vi "Drive Train.vi"   [LabVIEW 2018]
uses:
  <vilib>/Rock Robotics/SystemInterfaces/DIO/FPGA_DIOChannel.ctl
  <vilib>/Rock Robotics/SystemInterfaces/AI/FPGA_AIChannel.ctl
  <vilib>/Rock Robotics/WPI/ThirdParty/Sensors/navX/_TypeDefs/FRIC_navX_DeviceNumbersTypeDef.ctl
  <vilib>/Rock Robotics/WPI/ThirdParty/Phoenix-LabVIEW/Motor Controller/Controls/CTRE_Phoenix_MotorControl_NeutralMode.ctl
  <vilib>/Rock Robotics/WPI/Counter/WPI_CounterDigitalInputToDigitalSource.vi
  Times/Times Global.vi
  Drive Train Global.vi
types:
  T1 = typedef "FPGA_AIChannel.ctl" = enum8{"AI 0", "AI 1", "AI 2", "AI 3", "AI MXP 0", "AI MXP 1", "AI MXP 2", "AI MXP 3", "Invalid"}
  T2 = typedef "FPGA_DIOChannel.ctl" = enum8{"DIO 0", "DIO 1", "DIO 2", "DIO 3", "DIO 4", "DIO 5", "DIO 6", "DIO 7", "DIO 8", "DIO 9", "DIO MXP 0", "DIO MXP 1", "DIO MXP 2", "DIO MXP 3", "DIO MXP 4", "DIO MXP 5", "DIO MXP 6", "DIO MXP 7", "DIO MXP 8", "DIO MXP 9", "DIO MXP 10", "DIO MXP 11", "DIO MXP 12", "DIO MXP 13", "DIO MXP 14", "DIO MXP 15", "SPI Port CS1", "SPI Port CS2", "SPI Port CS3", "SPI Port MISO", "SPI Port MOSI", "Invalid"}
  T3 = typedef "CTRE_Phoenix_MotorControl_NeutralMode.ctl" = enum8{"EEPROMSetting", "Override to Coast", "Override to Brake"}
  T4 = typedef "WPI_MotorControlDeviceRef.ctl" = cluster{"DeviceStatus":errorcluster, "Type":T5, "PWM":cluster{"PWM Channel":T6, "DeadBand":T7}, "CAN":cluster{"Device Number":u8, "SetOutput VI Ref":variant, "GetOutput VI Ref":variant, "Enable VI Ref":variant, "Disable VI Ref":variant, "Data":variant}, "Invert":bool, "DIO PWM":cluster{"PWM \"Enable\" Channel":T6, "DIOChannel":T2, "PWM Rate":dbl}}
  T5 = typedef "WPI_MotorControlType.ctl" = enum16{"PWM", "CAN", "DIO PWM"}
  T6 = typedef "FPGA_DIOPWMChannel.ctl" = enum8{"PWM 0", "PWM 1", "PWM 2", "PWM 3", "PWM 4", "PWM 5", "PWM 6", "PWM 7", "PWM 8", "PWM 9", "PWM MXP 0", "PWM MXP 1", "PWM MXP 2", "PWM MXP 3", "PWM MXP 4", "PWM MXP 5", "PWM MXP 6", "PWM MXP 7", "PWM MXP 8", "PWM MXP 9", "Invalid"}
  T7 = typedef "WPI_PWMDeadband.ctl" = cluster{"Name":string, "maxPositivePwm":i32, "minPositivePwm":i32, "centerPwm":i32, "maxNegativePwm":i32, "minNegativePwm":i32, "angularRange":u16}
  T8 = typedef "WPI_DigitalInputDevRef.ctl" = cluster{"DevStatus":errorcluster, "DIO Channel":T2}
  T9 = typedef "WPI_PotentiometerDevRef.ctl" = cluster{"DevStatus":errorcluster, "Analog Channel":T1, "Invert Output":bool}
  T10 = typedef "FPGA_CounterEncoderSourceConvertionLVSourceType.ctl" = cluster{"DevStatus":errorcluster, "AnalogTriggerMode?":bool, "DigitalMode":cluster{"DIO Channel":T11}, "AnalogTriggerMode":cluster{"AnalogTriggerIndex":T12, "OutputType":T13}}
  T11 = typedef "FPGA_DIODigitalSourceChannel.ctl" = enum8{"DIO 0", "DIO 1", "DIO 2", "DIO 3", "DIO 4", "DIO 5", "DIO 6", "DIO 7", "DIO 8", "DIO 9", "DIO MXP 0", "DIO MXP 1", "DIO MXP 2", "DIO MXP 3", "DIO MXP 4", "DIO MXP 5", "DIO MXP 6", "DIO MXP 7", "DIO MXP 8", "DIO MXP 9", "DIO MXP 10", "DIO MXP 11", "DIO MXP 12", "DIO MXP 13", "DIO MXP 14", "DIO MXP 15", "SPI Port CS1", "SPI Port CS2", "SPI Port CS3", "SPI Port MISO", "SPI Port MOSI", "Disabled"}
  T12 = typedef "FPGA_AnalogTriggerIndex.ctl" = enum8{"Trig 0", "Trig 1", "Trig 2", "Trig 3", "Trig 4", "Trig 5", "Trig 6", "Trig 7", "Invalid"}
  T13 = typedef "FPGA_AnalogTriggerOutType.ctl" = enum16{"InWindow", "TriggerState", "Rising", "Falling"}
  T14 = typedef "WPI_EncoderDevRef.ctl" = cluster{"DevStatus":errorcluster, "EncoderIndex":T15, "CounterIndex":T16, "DistancePerCount":dbl, "Decoding Type":T17}
  T15 = typedef "FPGA_EncoderIdx.ctl" = enum8{"Enc 0", "Enc 1", "Enc 2", "Enc 3", "Enc 4", "Enc 5", "Enc 6", "Enc 7", "Invalid"}
  T16 = typedef "FPGA_CounterCtrSystemIndex.ctl" = enum8{"Ctr 0", "Ctr 1", "Ctr 2", "Ctr 3", "Ctr 4", "Ctr 5", "Ctr 6", "Ctr 7", "Invalid"}
  T17 = typedef "WPI_EncoderType.ctl" = enum16{"1x", "2x", "4x"}
  T18 = typedef "FRIC_navX_DeviceNumbersTypeDef.ctl" = enum16{"Dev0", "Dev1", "Dev2", "Dev3"}
  T19 = typedef "Control 2.ctl" = dbl
  T20 = cluster{"Rollover":dbl, "Yaw":dbl, "Cont Yaw":dbl}
  T21 = cluster{"FrontLeft":dbl, "FrontRight":dbl, "BackLeft":dbl, "BackRight":dbl}
  T22 = enum16{"Back Left", "Back Right", "Front Left", "Front Right"}
  T23 = enum16{"Autonomous Mode", "Field Oriented", "Robot Oriented", "Tank Mode"}
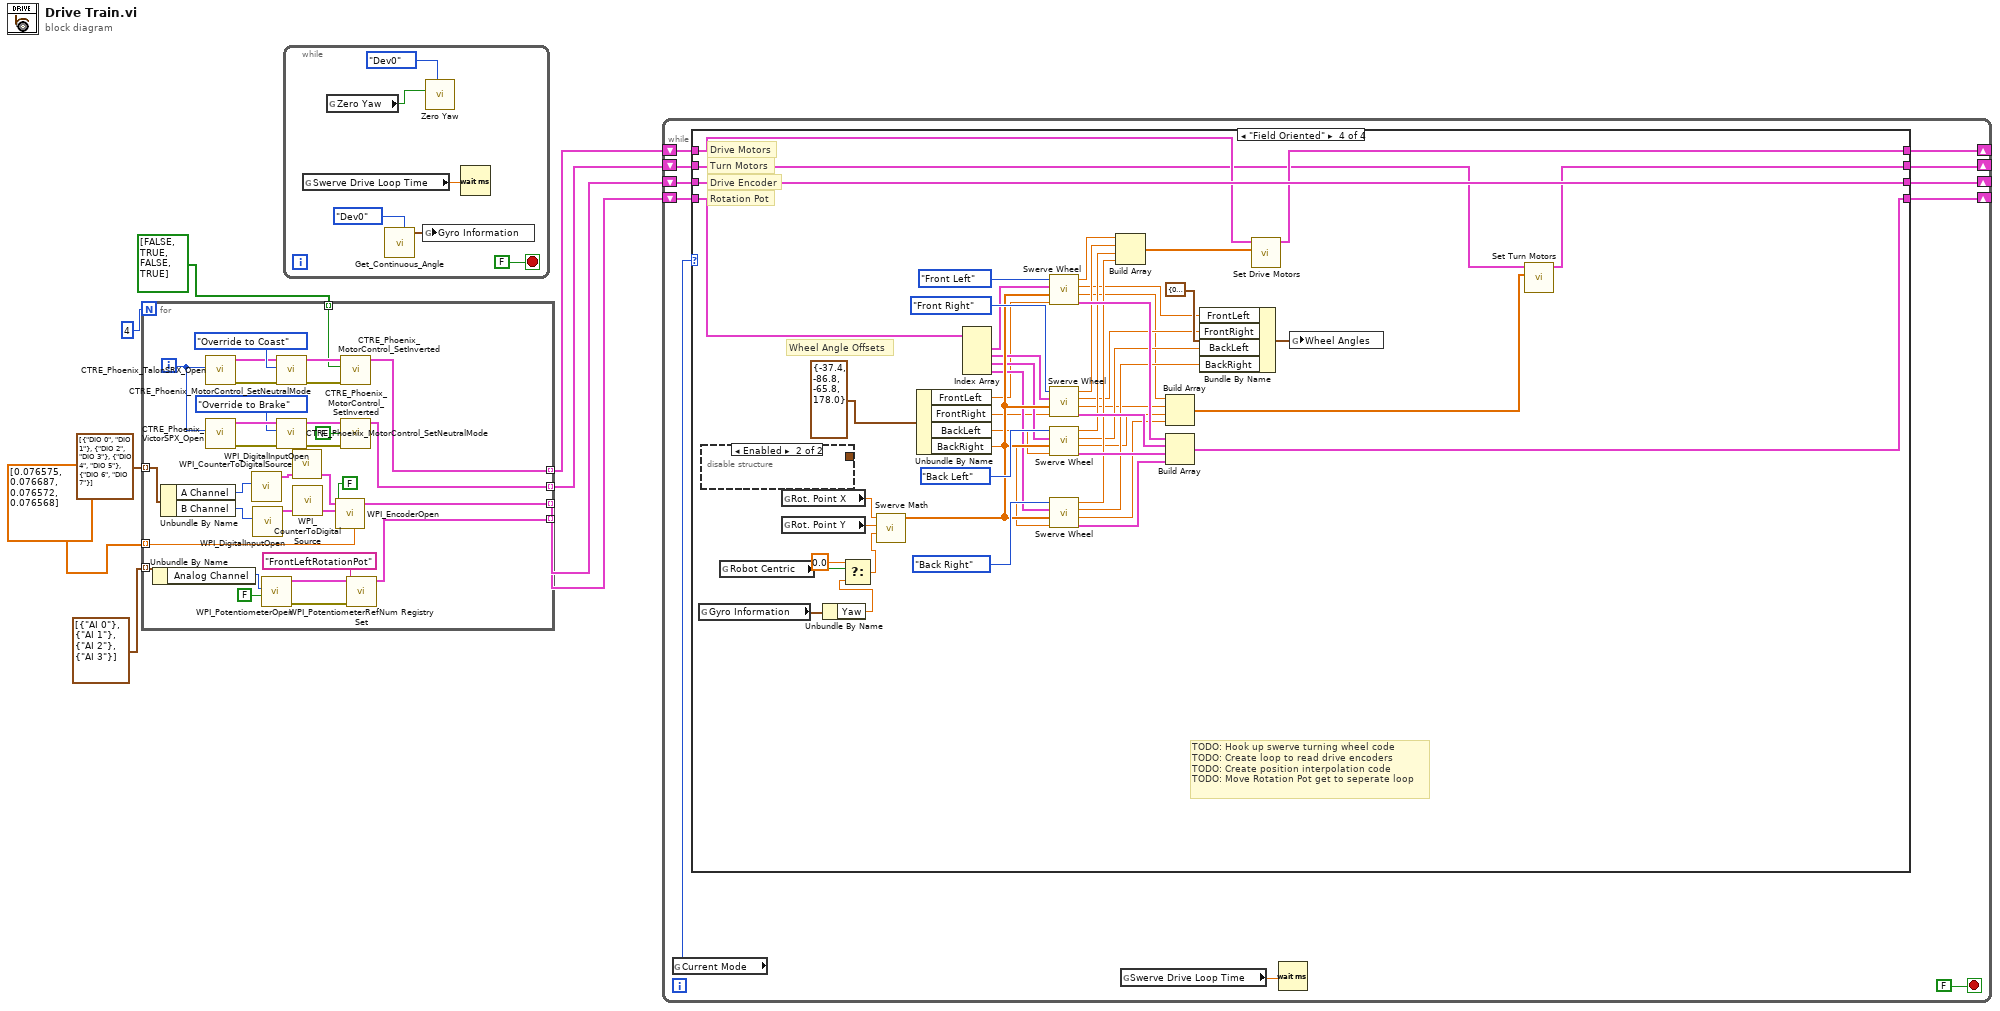
[diagram p0: block diagram]
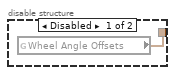
[diagram p5: hidden frame]
diagram:
  n1 = for {
    N: 4 -> [_]
    tunnel: cluster{"A Channel":T2, "B Channel":T2}[] [{"A Channel"=enum."DIO 0", "B Channel"=enum."DIO 1"}, {"A Channel"=enum."DIO 2", "B Channel"=enum."DIO 3"}, {"A Channel"=enum."DIO 4", "B Channel"=enum."DIO 5"}, {"A Channel"=enum."DIO 6", "B Channel"=enum."DIO 7"}] -> [w20] mode=indexing
    tunnel: cluster{"Analog Channel":T1}[] [{"Analog Channel"=enum."AI 0"}, {"Analog Channel"=enum."AI 1"}, {"Analog Channel"=enum."AI 2"}, {"Analog Channel"=enum."AI 3"}] -> [w17] mode=indexing
    tunnel: dbl[] [0.076575, 0.076687, 0.076572, 0.076568] -> [w15] mode=indexing
    tunnel: [w14] -> w5 mode=indexing
    tunnel: [w13] -> w4 mode=indexing
    tunnel: [w12] -> w3 mode=indexing
    tunnel: [w11] -> w2 mode=indexing
    tunnel: bool[] [FALSE, TRUE, FALSE, TRUE] -> [w10] mode=indexing
    i -> [w21]
    n2 = Unbundle By Name(w17) -> ("Analog Channel"=w16:T1)
    n3 = Unbundle By Name(w20) -> ("A Channel"=w19:T2, "B Channel"=w18:T2)
    n4 = call <vilib>:"CTRE_Phoenix_TalonSRX_Open.vi"("Device Number"=w21) -> ("error out"=w22:errorcluster, "CAN Talon SRX Ref"=w23:T4)  [unwired: 9 in]
    n5 = call <vilib>:"CTRE_Phoenix_VictorSPX_Open.vi"("Device Number"=w21) -> ("error out"=w32:errorcluster, "CAN Talon SRX Ref"=w31:T4)  [unwired: 9 in]
    n6 = call <vilib>:"WPI_DigitalInputOpen.vi"("DIO Channel"=w19) -> ("DigitalInputDevRef"=w39:T8)  [unwired: 1 in, 9 out]
    n7 = call <vilib>:"WPI_DigitalInputOpen.vi"("DIO Channel"=w18) -> ("DigitalInputDevRef"=w38:T8)  [unwired: 1 in, 9 out]
    n8 = call <vilib>:"WPI_PotentiometerOpen.vi"("Invert Output"=FALSE, "Analog Channel"=w16) -> ("error out"=w34:errorcluster, "PotDevRef"=w35:T9)  [unwired: 8 in]
    n9 = call <vilib>:"CTRE_Phoenix_MotorControl_SetNeutralMode.vi"("error in (no error)"=w22, "Motor Control Neutral Mode"=CTRE_Phoenix_MotorControl_NeutralMode."Override to Coast", "PhoenixMotorControlDevRef"=w23) -> ("error out"=w25:errorcluster, "PhoenixMotorControlDevRef"=w26:T4)  [unwired: 7 in]
    n10 = call <vilib>:"CTRE_Phoenix_MotorControl_SetNeutralMode.vi"("error in (no error)"=w32, "Motor Control Neutral Mode"=CTRE_Phoenix_MotorControl_NeutralMode."Override to Brake", "PhoenixMotorControlDevRef"=w31) -> ("error out"=w29:errorcluster, "PhoenixMotorControlDevRef"=w28:T4)  [unwired: 7 in]
    n11 = call-poly <vilib>:"WPI_CounterToDigitalSource.vi"("DigitalInputDevRef"=w39) -> ("Digital Source"=w40:T10)  [unwired: 6 out]
    n12 = call-poly <vilib>:"WPI_CounterToDigitalSource.vi"("DigitalInputDevRef"=w38) -> ("Digital Source"=w37:T10)  [unwired: 6 out]
    n13 = call <vilib>:"WPI_EncoderOpen.vi"("DistancePerCount"=w15, "Invert Direction (False)"=FALSE, "BSource"=w37, "ASource"=w40) -> ("EncoderDevRef"=w12:T14)  [unwired: 4 in, 3 out]
    n14 = call <vilib>:"CTRE_Phoenix_MotorControl_SetInverted.vi"("error in (no error)"=w25, "Invert?"=w10, "PhoenixMotorControlDevRef"=w26) -> ("PhoenixMotorControlDevRef"=w14:T4)  [unwired: 7 in, 1 out]
    n15 = call <vilib>:"CTRE_Phoenix_MotorControl_SetInverted.vi"("error in (no error)"=w29, "Invert?"=FALSE, "PhoenixMotorControlDevRef"=w28) -> ("PhoenixMotorControlDevRef"=w13:T4)  [unwired: 7 in, 1 out]
    n16 = call <vilib>:"WPI_PotentiometerRefNum Registry Set.vi"("error in (no error)"=w34, "refnum name"="FrontLeftRotationPot", "PotDevRef"=w35) -> ("PotDevRef"=w11:T9)  [unwired: 7 in, 1 out]
  }
  n17 = while {
    stop <- FALSE stop-if-true
    n18 = global read "Times Global.vi" "Swerve Drive Loop Time"() -> (w44:T19)
    n19 = global read "Drive Train Global.vi" "Zero Yaw"() -> (w43:bool)
    n20 = call <vilib>:"Get_Continuous_Angle.vi"("Device Number"=FRIC_navX_DeviceNumbersTypeDef."Dev0") -> ("Continuous Angle"=w45:T20)  [unwired: 10 in]
    n21 = global write "Drive Train Global.vi" "Gyro Information"(w45) -> ()
    n22 = call <vilib>:"Zero Yaw.vi"("Device Number"=FRIC_navX_DeviceNumbersTypeDef."Dev0", "Zero"=w43) -> ()  [unwired: 10 in]
    n23 = Wait (ms)(milliseconds to wait=w44) -> ()  [unwired: 1 out]
  }
  n24 = while {
    shift-right: [w51] -> _
    shift-left: w5 -> [w55]
    shift-right: [w50] -> _
    shift-left: w4 -> [w54]
    shift-right: [w49] -> _
    shift-left: w3 -> [w53]
    shift-right: [w48] -> _
    shift-left: w2 -> [w52]
    stop <- FALSE stop-if-true
    n25 = global read "Drive Train Global.vi" "Current Mode"() -> (w56:T23)
    n26 = case shown="\"Field Oriented\"" w56 {
      tunnel: w55 -> [w62 w66 w70 w94]
      tunnel: w54 -> [w61 w65 w69 w82]
      tunnel: w53 -> [w60 w64 w68 w114]
      tunnel: w52 -> [w59 w63 w67 w105]
      tunnel: [w62 w66 w70 w93] -> w51
      tunnel: [w61 w65 w69 w81] -> w50
      tunnel: [w60 w64 w68 w114] -> w49
      tunnel: [w59 w63 w67 w104] -> w48
      frame "Autonomous Mode", Default {
        # "Rotation Pot"
        # "Drive Encoder"
        # "Turn Motors"
        # "Drive Motors"
      }
      frame "Robot Oriented" {
        # "Rotation Pot"
        # "Drive Encoder"
        # "Turn Motors"
        # "Drive Motors"
      }
      frame "Tank Mode" {
        # "Rotation Pot"
        # "Drive Encoder"
        # "Turn Motors"
        # "Drive Motors"
      }
      frame "Field Oriented" {
        # "Wheel Angle Offsets"
        # "TODO: Hook up swerve turning wheel code\nTODO: Create loop to read drive encoders\nTODO: Create position interpolation code\nTODO: Move Rotation Pot get to seperate loop"
        # "Rotation Pot"
        # "Drive Encoder"
        # "Turn Motors"
        # "Drive Motors"
        n27 = global read "Drive Train Global.vi" "Gyro Information"() -> (w112:T20)
        n28 = disable-structure shown="Enabled" {
          disable-tunnel: [w119 _] -> _
          frame Disabled {
            n29 = global read "Drive Train Global.vi" "Wheel Angle Offsets"() -> (w119:T21)
          }
          frame Enabled {
          }
        }
        n30 = global read "Drive Train Global.vi" "Robot Centric"() -> (w74:bool)
        n31 = global read "Drive Train Global.vi" "Rot. Point X"() -> (w111:dbl)
        n32 = global read "Drive Train Global.vi" "Rot. Point Y"() -> (w110:dbl)
        n33 = Unbundle By Name(w112) -> ("Yaw"=w72:dbl)
        n34 = Select(t=0.0, s=w74, f=w72) -> (s? t:f=w75:dbl)
        n35 = call "Swerve Math.vi"("Yaw"=w75, "Rot. Point Y"=w110, "Rot. Point X"=w111) -> ("Swerve Math Ouput"=w113:dbl[])  [unwired: 8 in]
        n36 = Unbundle By Name(T21 {"FrontLeft"=-37.4, "FrontRight"=-86.8, "BackLeft"=-65.8, "BackRight"=178.0} ("Wheel Angle Offsets")) -> ("FrontLeft"=w79:dbl, "FrontRight"=w78:dbl, "BackLeft"=w77:dbl, "BackRight"=w76:dbl)
        n37 = Index Array(array=w105) -> (element #1=w109:T9, element #2=w108:T9, element #3=w107:T9, element #4=w106:T9)  [unwired: 4 in]
        n38 = call "Swerve Wheel.vi"("Wheel Angle Offset"=w79, "Inputs"=w113, "Pot Ref In"=w109, "Wheel"=T22."Front Left") -> ("Pot Ref Out"=w100:T9, "Motor Output"=w86:dbl, "Wheel Angle"=w91:dbl, "Speed"=w99:dbl)  [unwired: 4 in]
        n39 = call "Swerve Wheel.vi"("Wheel Angle Offset"=w78, "Inputs"=w113, "Pot Ref In"=w108, "Wheel"=T22."Front Right") -> ("Pot Ref Out"=w101:T9, "Motor Output"=w85:dbl, "Wheel Angle"=w90:dbl, "Speed"=w98:dbl)  [unwired: 4 in]
        n40 = call "Swerve Wheel.vi"("Wheel Angle Offset"=w77, "Inputs"=w113, "Pot Ref In"=w107, "Wheel"=T22."Back Left") -> ("Pot Ref Out"=w102:T9, "Motor Output"=w84:dbl, "Wheel Angle"=w89:dbl, "Speed"=w97:dbl)  [unwired: 4 in]
        n41 = call "Swerve Wheel.vi"("Wheel Angle Offset"=w76, "Inputs"=w113, "Pot Ref In"=w106, "Wheel"=T22."Back Right") -> ("Pot Ref Out"=w103:T9, "Motor Output"=w83:dbl, "Wheel Angle"=w88:dbl, "Speed"=w96:dbl)  [unwired: 4 in]
        n42 = Build Array(w99, w98, w97, w96) -> (w95:dbl[])
        n43 = Build Array(w86, w85, w84, w83) -> (w80:dbl[])
        n44 = Build Array(w100, w101, w102, w103) -> (w104:T9[])
        n45 = Bundle By Name(cluster=T21 {"FrontLeft"=0.0, "FrontRight"=0.0, "BackLeft"=0.0, "BackRight"=0.0} ("Wheel Angles"), "FrontLeft"=w91, "FrontRight"=w90, "BackLeft"=w89, "BackRight"=w88) -> (w87:T21)
        n46 = call "Set Drive Motors.vi"("appended array"=w95, "Motors In"=w94) -> ("Motors Out"=w93:T4[])  [unwired: 9 in]
        n47 = global write "Drive Train Global.vi" "Wheel Angles"(w87) -> ()
        n48 = call "Set Turn Motors.vi"("appended array"=w80, "Motors In"=w82) -> ("Motors Out"=w81:T4[])  [unwired: 9 in]
      }
    }
    n49 = global read "Times Global.vi" "Swerve Drive Loop Time"() -> (w57:T19)
    n50 = Wait (ms)(milliseconds to wait=w57) -> ()  [unwired: 1 out]
  }
